vi "Encode Pixel.vi"(8 "3 Bits":bool[](array[boolean]), 9 "B":u8(slide) scale=0.0..255.0, 10 "G":u8(slide) scale=0.0..255.0, 11 "R":u8(slide) scale=0.0..255.0) -> (1 "B 2":u8(slide) scale=0.0..255.0, 2 "G 2":u8(slide) scale=0.0..255.0, 3 "R 2":u8(slide) scale=0.0..255.0)   [LabVIEW 2020]
panel:
  out "Avg 2":i32(slide) scale=0.0..255.0
  out "New Color":u32(colorbox)
  out "Avg":i32(slide) scale=0.0..255.0
  out "Source Color":u32(colorbox)
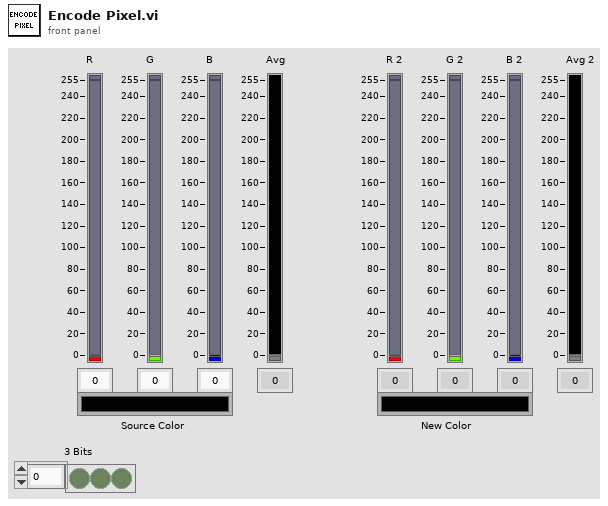
[diagram p1: front panel]
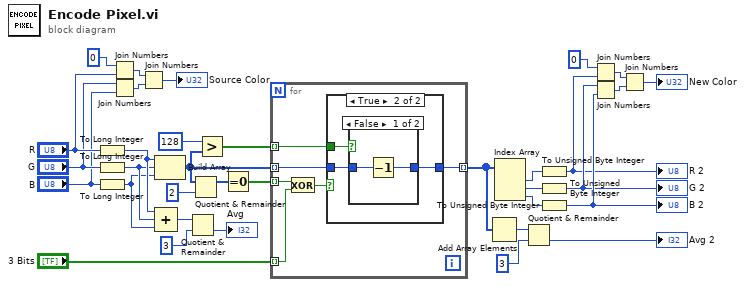
[diagram p0: block diagram]
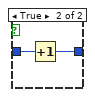
[diagram p3: hidden frame]
diagram:
  n1 = To Long Integer(number="R") -> (32bit integer=w32:i32)
  n2 = To Long Integer(number="G") -> (32bit integer=w31:i32)
  n3 = To Long Integer(number="B") -> (32bit integer=w30:i32)
  n4 = Join Numbers(hi=u8 0, lo="R") -> ((hi.lo)=w26:u16)
  n5 = Join Numbers(hi="G", lo="B") -> ((hi.lo)=w25:u16)
  n6 = Join Numbers(hi=w26, lo=w25) -> ((hi.lo)=→"Source Color":u32)
  n7 = Build Array(w32, w31, w30) -> (w7:i32[])
  n8 = Compound Arithmetic op=ADD(w32, w31, w30) -> (w34:i32)
  n9 = Quotient & Remainder(x=w34, y=3) -> (floor(x/y)=→"Avg":i32)  [unwired: 1 out]
  n10 = Quotient & Remainder(x=w7, y=2) -> (x-y*floor(x/y)=w9:i32[])  [unwired: 1 out]
  n11 = Greater?(x=128, y=w7) -> (0:w5:bool[])
  n12 = Equal To 0?(x=w9) -> (x = 0?=w8:bool[])
  n13 = for {
    tunnel: "3 Bits" -> [w39] mode=indexing
    tunnel: w7 -> [w37] mode=indexing
    tunnel: w8 -> [w40] mode=indexing
    tunnel: w5 -> [w35] mode=indexing
    tunnel: [w36] -> w1 mode=indexing
    n14 = Exclusive Or(1:w39, 2:w40) -> (0:w38:bool)
    n15 = case shown="True" w38 {
      tunnel: w37 -> [w41 w43]
      tunnel: [w41 w42] -> w36
      tunnel: w35 -> [_ w44]
      frame False {
      }
      frame True {
        n16 = case shown="False" w44 {
          tunnel: w43 -> [w46 w48]
          tunnel: [w45 w47] -> w42
          frame False {
            n17 = Decrement(x=w46) -> (x-1=w45:i32)
          }
          frame True {
            n18 = Increment(x=w48) -> (x+1=w47:i32)
          }
        }
      }
    }
  }
  n19 = Add Array Elements(numeric array=w1) -> (sum=w29:i32)
  n20 = Index Array(array=w1) -> (element #1=w3:i32, element #2=w4:i32, element #3=w2:i32)  [unwired: 3 in]
  n21 = Quotient & Remainder(x=w29, y=3) -> (floor(x/y)=→"Avg 2":i32)  [unwired: 1 out]
  n22 = To Unsigned Byte Integer(number=w3) -> (unsigned 8bit integer=w14:u8)
  "R 2" <- w14
  n23 = To Unsigned Byte Integer(number=w4) -> (unsigned 8bit integer=w15:u8)
  "G 2" <- w15
  n24 = To Unsigned Byte Integer(number=w2) -> (unsigned 8bit integer=w16:u8)
  "B 2" <- w16
  n25 = Join Numbers(hi=u8 0, lo=w14) -> ((hi.lo)=w19:u16)
  n26 = Join Numbers(hi=w15, lo=w16) -> ((hi.lo)=w18:u16)
  n27 = Join Numbers(hi=w19, lo=w18) -> ((hi.lo)=→"New Color":u32)
